vi "test-profiled-PID.vi"() -> (3 "Test Passed 0":bool)   [LabVIEW 2019]
uses:
  <vilib>/Rock Robotics/WPI/ThirdParty/JAS_Junk/TrajLib/ProfiledPIDController_NewPeriod.vi
  <vilib>/Rock Robotics/WPI/ThirdParty/JAS_Junk/TrajLib/TrapProfState_New.vi
  <vilib>/Rock Robotics/WPI/ThirdParty/JAS_Junk/TrajLib/ProfiledPIDController_Reset.vi
  <vilib>/Rock Robotics/WPI/ThirdParty/JAS_Junk/TrajLib/PIDController_Calculate_SP_PV.vi
  <vilib>/Rock Robotics/WPI/ThirdParty/JAS_Junk/TrajLib/TrapProfile_New.vi
  <vilib>/Rock Robotics/WPI/ThirdParty/JAS_Junk/TrajLib/ProfiledPIDController_GetPeriod.vi
  <vilib>/Rock Robotics/WPI/ThirdParty/JAS_Junk/TrajLib/TrapProfile_Calculate.vi
  <vilib>/Rock Robotics/WPI/ThirdParty/JAS_Junk/TrajLib/ControllerUtil_GetModulusError.vi
  <vilib>/Rock Robotics/WPI/ThirdParty/JAS_Junk/TrajLib/PIDController_NewPeriod.vi
  <vilib>/Rock Robotics/SystemInterfaces/NetworkCommunication/NetComm_UsageReport_report.vi
  <vilib>/Rock Robotics/WPI/ThirdParty/JAS_Junk/TrajLib/PIDController_Reset.vi
  <vilib>/Rock Robotics/WPI/ThirdParty/JAS_Junk/TrajLib/PIDController_SetSetpoint.vi
  <vilib>/Rock Robotics/WPI/ThirdParty/JAS_Junk/TrajLib/PIDController_Calculate_PV.vi
  <vilib>/Rock Robotics/WPI/ThirdParty/JAS_Junk/TrajLib/TrapProfile_ShouldFlipAcceleration.vi
  <vilib>/Rock Robotics/WPI/ThirdParty/JAS_Junk/TrajLib/TrapProfile_Direct.vi
  <vilib>/Rock Robotics/WPI/ThirdParty/JAS_Junk/TrajLib/PIDController_GetPeriod.vi
  <vilib>/Rock Robotics/WPI/ThirdParty/JAS_Junk/TrajLib/Util_LibraryGlobals.vi
  <vilib>/Rock Robotics/WPI/ThirdParty/JAS_Junk/TrajLib/Trajectory_Library.lvlib
panel:
  out "T0 -- Output approx 0":dbl
  # "Profiled PID"
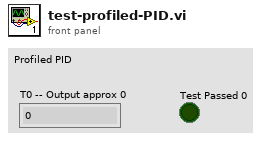
[diagram p1: front panel]
types:
  T1 = typedef "Trajectory_Library.lvlib/TRAPEZOID_PROFILE_CONSTRAINT.ctl" = cluster{"MaxVelocity":dbl, "MaxAcceleration":dbl}
  T2 = typedef "Trajectory_Library.lvlib/PROFILED_PID_CONTROLLER.ctl" = cluster{"Controller":T3, "Goal":T4, "Setpoint":T4, "Constraint":T1}
  T3 = typedef "Trajectory_Library.lvlib/PID_CONTROLLER.ctl" = cluster{"Kp":dbl, "Ki":dbl, "Kd":dbl, "Period":dbl, "Max_Integral":dbl, "Min_Integral":dbl, "Max_Input":dbl, "Min_Input":dbl, "Continuous":bool, "PositionError":dbl, "VelocityError":dbl, "PrevError":dbl, "TotalError":dbl, "PositionTolerance":dbl, "VelocityTolerance":dbl, "SetPoint":dbl, "Kf":dbl, "Prev_Deriv":dbl, "Prev_Deriv 2":dbl, "DerivativeFilter":bool, "Min_Output":dbl, "Max_Output":dbl, "Prev_F_P":dbl, "Prev_F_P_2":dbl, "AntiWindupActive":bool, "Measurement":dbl}
  T4 = typedef "Trajectory_Library.lvlib/TRAPEZOID_PROFILE_STATE.ctl" = cluster{"Position":dbl, "Velocity":dbl}
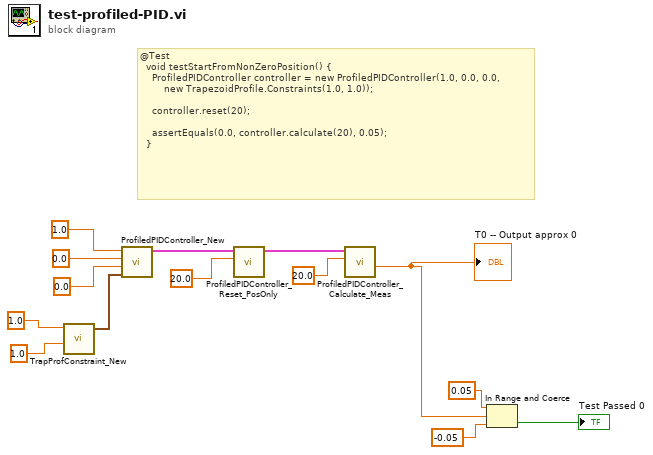
[diagram p0: block diagram]
diagram:
  # "@Test\n  void testStartFromNonZeroPosition() {\n    ProfiledPIDController controller = new ProfiledPIDController(1.0, 0.0, 0.0,\n        new TrapezoidProfile.Constraints(1.0, 1.0));\n\n    controller.reset(20);\n\n    assertEquals(0.0, controller.calculate(20), 0.05);\n  }"
  n1 = call <vilib>:"TrapProfConstraint_New.vi"("Max Accel"=1.0, "Max Speed (M/S)"=1.0 ("Max Accel")) -> ("TRAPEZOID_PROFILE_CONSTRAINT"=w9:T1)  [unwired: 9 in]
  n2 = call <vilib>:"ProfiledPIDController_New.vi"("Constraints"=w9, "Kd"=0.0 ("Kp"), "Ki"=0.0 ("Kp"), "Kp"=1.0) -> ("PROFILED_PID_CONTROLLER"=w7:T2)  [unwired: 7 in]
  n3 = call <vilib>:"ProfiledPIDController_Reset_PosOnly.vi"("Position"=20.0, "in PROFILED_PID_CONTROLLER"=w7) -> ("out PROFILED_PID_CONTROLLER"=w6:T2)  [unwired: 9 in]
  n4 = call <vilib>:"ProfiledPIDController_Calculate_Meas.vi"("PV-Measurement"=20.0, "in PROFILED_PID_CONTROLLER"=w6) -> ("CO-ControlOutput"=w1:dbl)  [unwired: 8 in, 1 out]
  "T0 -- Output approx 0" <- w1
  n5 = In Range and Coerce(upper limit=0.05, x=w1, lower limit=-0.05) -> (In Range?=→"Test Passed 0":bool)  [unwired: 1 out]
